vi "Set State.vi"(8 "error in (no error)":errorcluster, 10 "Output":T1, 11 "Inst.RP100 in":refnum<class "Inst.RP100.lvclass">) -> (0 "error out":errorcluster, 3 "Inst.RP100 out":refnum<class "Inst.RP100.lvclass">)   [LabVIEW 2019, in "Inst.RP100.lvclass"]
doc: "Set the output <b>Level</b> with <b>Slew</b> rate on the selected <b>Output Channel</b>"
uses:
  Inst.RP100.lvclass
  Typedefs/State--Enum.ctl
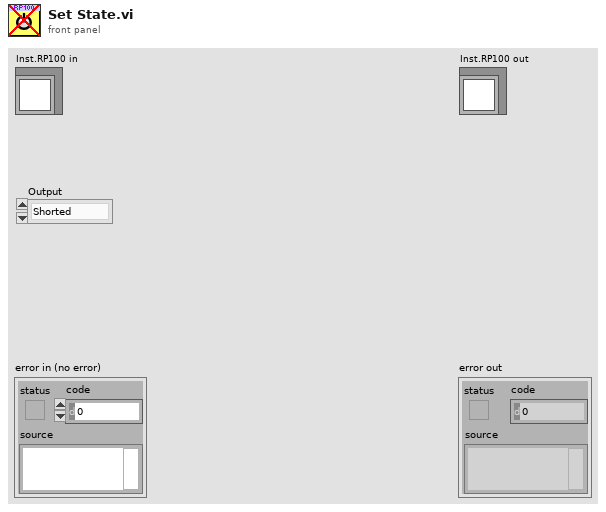
[diagram p1: front panel]
types:
  T1 = typedef "Inst.RP100.lvclass/State--Enum.ctl" = enum16{"Shorted", "Enabled"}
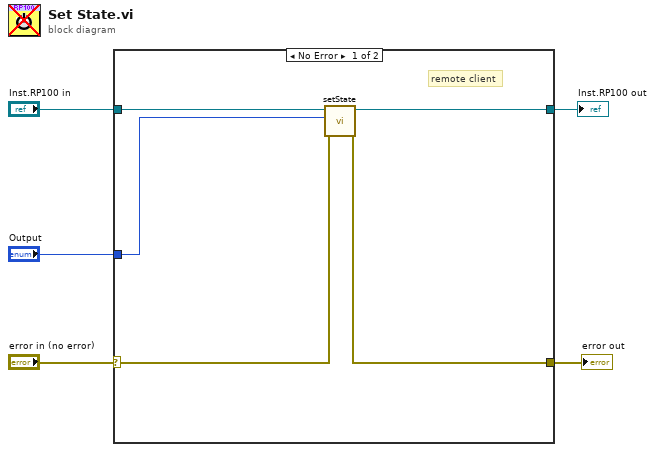
[diagram p0: block diagram]
diagram:
  n1 = case shown="No Error" "error in (no error)" {
    selector: "error in (no error)" -> [w8 w12]
    tunnel: [w7 w12] -> w4
    tunnel: "Output" -> [w10 _]
    tunnel: "Inst.RP100 in" -> [w9 w11]
    tunnel: [w6 w11] -> w1
    frame No Error {
      # "remote client"
      n2 = call-dynamic "setState.vi"("error in (no error)"=w8, "Output"=w10, "Inst.RP100 in"=w9) -> ("error out"=w7:errorcluster, "Inst.RP100 out"=w6:refnum<class "Inst.RP100.lvclass">)  [unwired: 7 in]
    }
    frame Error {
    }
  }
  "error out" <- w4
  "Inst.RP100 out" <- w1
